vi "same_loop+keyboard.vi"() -> ()   [LabVIEW 2015]
doc: "Very simple example showing how to use the base VIs to control the AR Drone and receive and display navigation data."
uses:
  <vilib>/LVH/AR Drone Toolkit/Type Defs/AR Drone Resource.ctl
  <vilib>/LVH/AR Drone Toolkit/Decode NavData/Typedefs/NavData Demo.ctl
  video_global.vi
  <vilib>/Utility/inputDevices.llb/closeKeyboard.vi
  <vilib>/LVH/AR Drone Toolkit/AR Drone.lvlib
panel:
  out "Final controls":cluster{dbl, dbl, dbl, dbl}
  in  "double precision float":cluster{dbl, dbl, dbl, dbl}
  in  "Numeric 2":dbl
  in  "Stop snap":bool
  in  "Grab photo":bool
  in  "Auto-Adjust":bool
  out "Battery Remaining 2":dbl(slide) scale=0.0..100.0
  out "NavData Out 2":T1
  out "Video Stream":picture
  out "AR Drone Resource":T2={"UDP Control Connection"=refnum, "UDP NavData Connection"=refnum, "UDP Video Connection (Drone 1.0)"=refnum, "TCP Video Connection (Drone 2.0)"=refnum, "TCP Control Port Connection"=refnum, "Drone IP address"="192.168.1.1", "Drone Command Port"=5556, "Drone NavData Port"=5554, "Drone Vid Stream Port"=5555, "Drone TCP Control Port"=5559, "Home IP address"="192.168.1.2", "Home Command Port"=56828, "Home NavData Port"=56829, "Home Vid Stream Port"=56830, "Drone Version"=0, "Drone Index"=0, "Command Sequence"=1}
  out "Numeric":i32
  out "x > y?":bool
  in  "Stop connection":bool
  in  "Emergency Landing":bool
  in  "Take Off/Land":bool
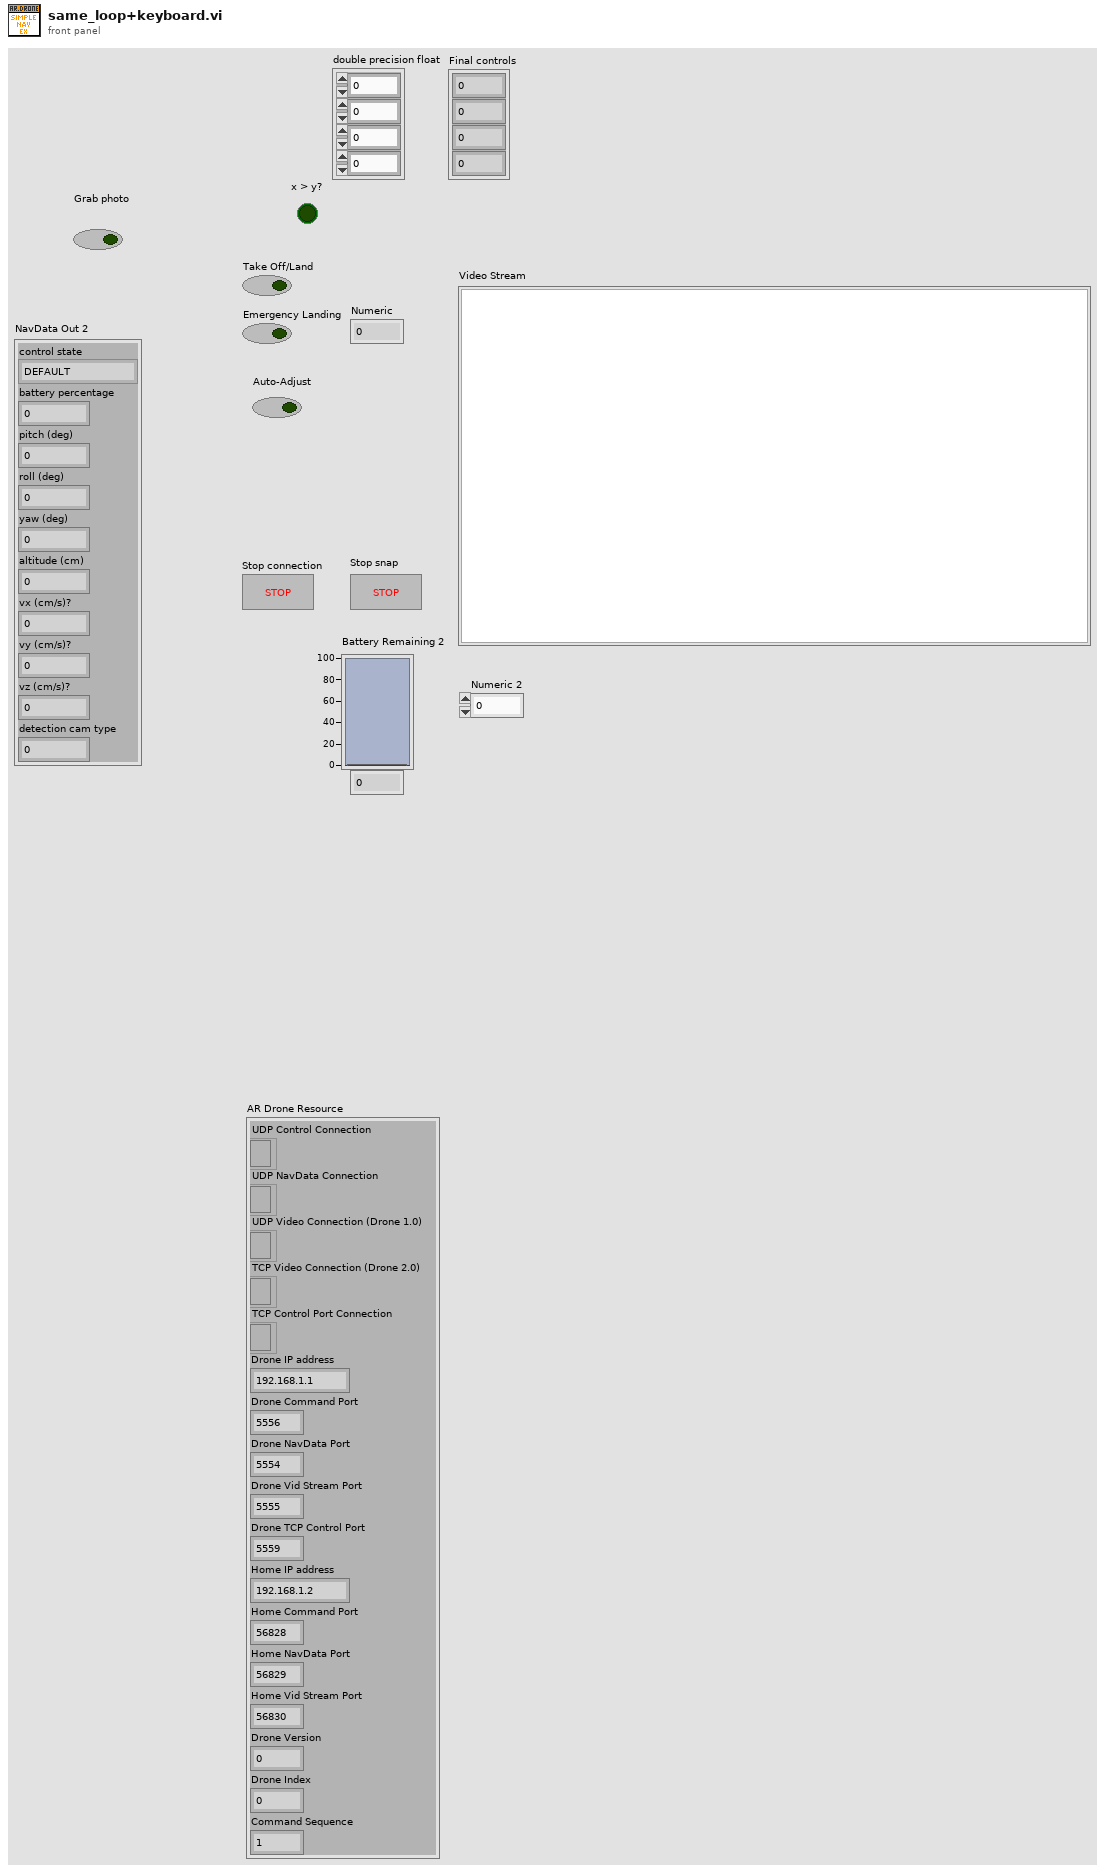
[diagram p1: front panel]
types:
  T1 = typedef "AR Drone.lvlib/NavData Demo.ctl" = cluster{"control state":enum32{"DEFAULT", "INIT", "LANDING", "FLYING", "HOVERING", "TEST", "TRANS_TAKEOFF", "TRANS_GOTOFIX", "TRANS_LANDING"}, "battery percentage":u32, "pitch (deg)":sgl, "roll (deg)":sgl, "yaw (deg)":sgl, "altitude (cm)":u32, "vx (cm/s)?":sgl, "vy (cm/s)?":sgl, "vz (cm/s)?":sgl, "detection cam type":u32}
  T2 = typedef "AR Drone.lvlib/AR Drone Resource.ctl" = cluster{"UDP Control Connection":refnum<k16>, "UDP NavData Connection":refnum<k16>, "UDP Video Connection (Drone 1.0)":refnum<k16>, "TCP Video Connection (Drone 2.0)":refnum<k5>, "TCP Control Port Connection":refnum<k5>, "Drone IP address":string, "Drone Command Port":u16, "Drone NavData Port":u16, "Drone Vid Stream Port":u16, "Drone TCP Control Port":u16, "Home IP address":string, "Home Command Port":u16, "Home NavData Port":u16, "Home Vid Stream Port":u16, "Drone Version":i32, "Drone Index":i32, "Command Sequence":i32}
  T3 = cluster{"Drone IP address":string, "Home IP address":string, "Flight Mode":enum8{"OUTDOOR MODE", "INDOOR MODE"}, "Mounted Hull":enum8{"OUTDOOR HULL", "INDOOR HULL"}, "Video Camera":u8, "Max Altitude (m)":sgl, "Max Pitch and Roll Angle (deg)":sgl, "Max Vertical Speed (m/s)":sgl, "Max Yaw Speed (deg/s)":sgl}
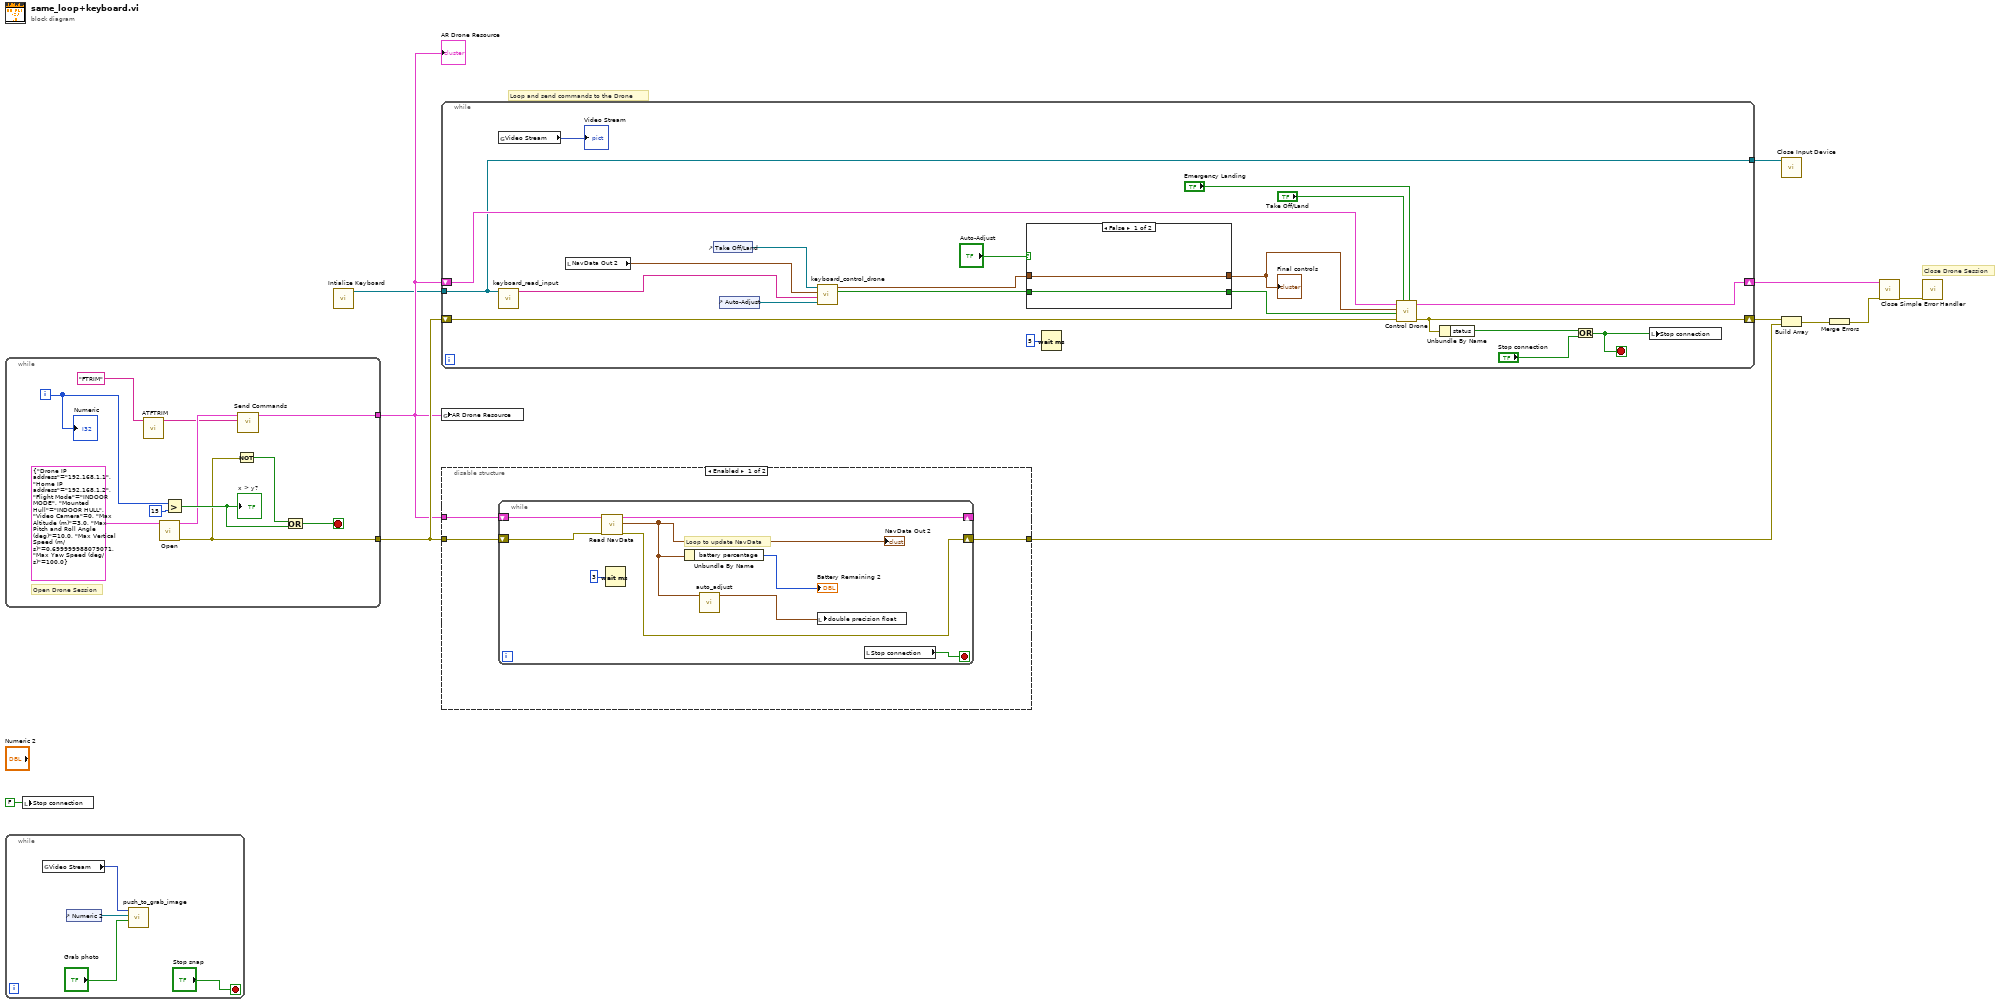
[diagram p0: block diagram]
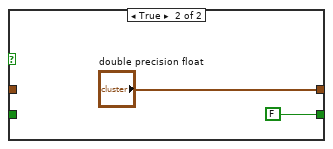
[diagram p3: hidden frame]
diagram:
  # "Close Drone Session"
  # "Loop and send commands to the Drone"
  n1 = while {
    tunnel: [w12] -> w4
    tunnel: [w16] -> w5
    i -> [w21]
    stop <- w17 stop-if-true
    # "Open Drone Session"
    n2 = call <vilib>:"ATFTRIM.vi"("Command String In"="FTRIM") -> ("Command String out"=w13:string)  [unwired: 12 in, 2 out]
    n3 = call <vilib>:"Open.vi"("Setup Parameters"=T3 {"Drone IP address"="192.168.1.1", "Home IP address"="192.168.1.2", "Flight Mode"=enum."INDOOR MODE", "Mounted Hull"=enum."INDOOR HULL", "Video Camera"=0, "Max Altitude (m)"=3.0, "Max Pitch and Roll Angle (deg)"=10.0, "Max Vertical Speed (m/s)"=0.7, "Max Yaw Speed (deg/s)"=100.0}) -> ("error out"=w16:errorcluster, "AR Drone Resource"=w14:T2)  [unwired: 9 in]
    n4 = Greater?(x=w21, y=15) -> (0:w18:bool)
    "x > y?" <- w18
    n5 = Not(x=w16) -> (.not. x?=w19:bool)
    n6 = call <vilib>:"Send Commands.vi"("Command String"=w13, "AR Drone Resource"=w14) -> ("AR Drone Resource Out"=w12:T2)  [unwired: 6 in, 1 out]
    n7 = Or(x=w19, y=w18) -> (x .or. y?=w17:bool)
    "Numeric" <- w21
  }
  "AR Drone Resource" <- w4
  n8 = while {
    stop <- "Stop snap" stop-if-true
    n9 = global read "video_global.vi" "Video Stream"() -> (w26:picture)
    n10 = control-ref of="Numeric 2"() -> (w23:refnum<vi>)
    n11 = call "push_to_grab_image.vi"("Boolean 2"="Grab photo", "DigNum Refnum"=w23, "picture"=w26) -> ()  [unwired: 7 in, 1 out]
  }
  n12 = local write "Stop connection"(FALSE) -> ()
  n13 = call <vilib>:"Intialize Keyboard.vi"() -> ("device ID"=w3:refnum<k1>)  [unwired: 10 in, 1 out]
  n14 = while {
    shift-right: [w45] -> w11
    shift-left: w4 -> [w40]
    shift-right: [w42] -> w9
    shift-left: w5 -> [w39]
    tunnel: w3 -> [w38]
    tunnel: [w38] -> w2
    stop <- w41 stop-if-true
    n15 = global read "video_global.vi" "Video Stream"() -> (→"Video Stream":picture)
    n16 = call "keyboard_read_input.vi"("device ID"=w38) -> ("resulting string"=w34:string)  [unwired: 10 in]
    n17 = local read "NavData Out 2"() -> (w27:T1)
    n18 = control-ref of="Take Off/Land"() -> (w35:refnum<vi>)
    n19 = control-ref of="Auto-Adjust"() -> (w30:refnum<vi>)
    n20 = call "keyboard_control_drone.vi"("Auto_mode"=w30, "resulting string"=w34, "NavData Out 2"=w27, "Take/off"=w35) -> ("Hover"=w29:bool, "Cluster"=w33:cluster{i32, i32, i32, i32})  [unwired: 6 in]
    n21 = case shown="False" "Auto-Adjust" {
      tunnel: [w49 "double precision float"] -> w36
      tunnel: w33 -> [w49 _]
      tunnel: w29 -> [w48 _]
      tunnel: [w48 FALSE] -> w28
      frame False {
      }
      frame True {
      }
    }
    "Final controls" <- w36
    n22 = Wait (ms)(milliseconds to wait=u32 5) -> ()  [unwired: 1 out]
    n23 = call <vilib>:"Control Drone.vi"("Emergency Landing"="Emergency Landing", "Takeoff/Land"="Take Off/Land", "error in (no error)"=w39, "Hover"=w28, "Control Cluster"=w36, "AR Drone Resource"=w40) -> ("error out"=w42:errorcluster, "AR Drone Resource Out"=w45:T2)  [unwired: 4 in]
    n24 = Unbundle By Name(w42) -> ("status"=w43:bool)
    n25 = Or(x=w43, y="Stop connection") -> (x .or. y?=w41:bool)
    n26 = local write "Stop connection"(w41) -> ()
  }
  n27 = global write "video_global.vi" "AR Drone Resource"(w4) -> ()
  n28 = disable-structure shown="Enabled" {
    disable-tunnel: [w54 _] -> w10
    disable-tunnel: w5 -> [w53 _]
    disable-tunnel: w4 -> [w52 _]
    frame Enabled {
      n29 = while {
        shift-right: [w59] -> _
        shift-left: w52 -> [w61]
        shift-right: [w58] -> w54
        shift-left: w53 -> [w60]
        stop <- w63 stop-if-true
        # "Loop to update NavData"
        n30 = call <vilib>:"Read NavData.vi"("error in (no error)"=w60, "AR Drone Resource"=w61) -> ("error out"=w58:errorcluster, "NavData Out"=w57:T1, "AR Drone Resource Out"=w59:T2)  [unwired: 7 in]
        "NavData Out 2" <- w57
        n31 = Wait (ms)(milliseconds to wait=u32 3) -> ()  [unwired: 1 out]
        n32 = Unbundle By Name(w57) -> ("battery percentage"=→"Battery Remaining 2":u32)
        n33 = call "auto_adjust.vi"("NavData Out 2"=w57) -> ("output cluster"=w56:cluster{"Change amount\n":dbl, dbl, i32, i32})  [unwired: 10 in]
        n34 = local write "double precision float"(w56) -> ()
        n35 = local read "Stop connection"() -> (w63:bool)
      }
    }
    frame Disabled {
    }
  }
  n36 = call-poly <vilib>:"Close Input Device.vi"("device ID"=w2) -> ()  [unwired: 9 in, 1 out]
  n37 = Build Array(w9, w10) -> (w6:errorcluster[])
  n38 = Merge Errors(w6) -> (w8:errorcluster)
  n39 = call <vilib>:"Close.vi"("error in (no error)"=w8, "AR Drone Resource"=w11) -> ("error out"=w7:errorcluster)  [unwired: 9 in]
  n40 = call <vilib>:"Simple Error Handler.vi"("error in (no error)"=w7) -> ()  [unwired: 4 in, 5 out]
